vi "Save Preset.vi"(5 "No Oxy?":bool, 6 "Dump Stat":T2, 7 "Preset Name":string, 8 "error in (no error)":errorcluster, 9 "Levels Available":i32, 10 "Levels":T3, 11 "Config":T1) -> (0 "error out":errorcluster, 3 "Config out":T1)   [LabVIEW 2023]
uses:
  <vilib>/Utility/config.llb/Config Data RefNum.ctl
  CTLs/Dump Stat.ctl
  <vilib>/Utility/config.llb/Write Key (I32).vi
  <vilib>/Utility/config.llb/NI_LVConfig.lvlib
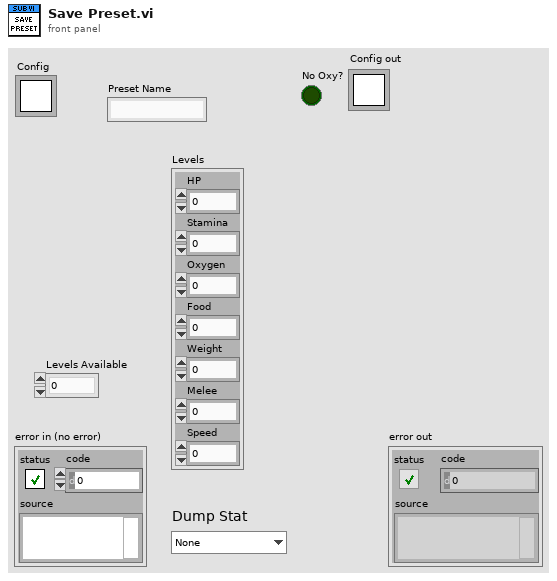
[diagram p1: front panel]
types:
  T1 = typedef "NI_LVConfig.lvlib/Config Data RefNum.ctl" = refnum<k1>
  T2 = typedef "Dump Stat.ctl" = enum16{"None", "HP", "Stamina", "Oxygen", "Food", "Weight", "Melee", "Speed"}
  T3 = cluster{"HP":i32, "Stamina":i32, "Oxygen":i32, "Food":i32, "Weight":i32, "Melee":i32, "Speed":i32}
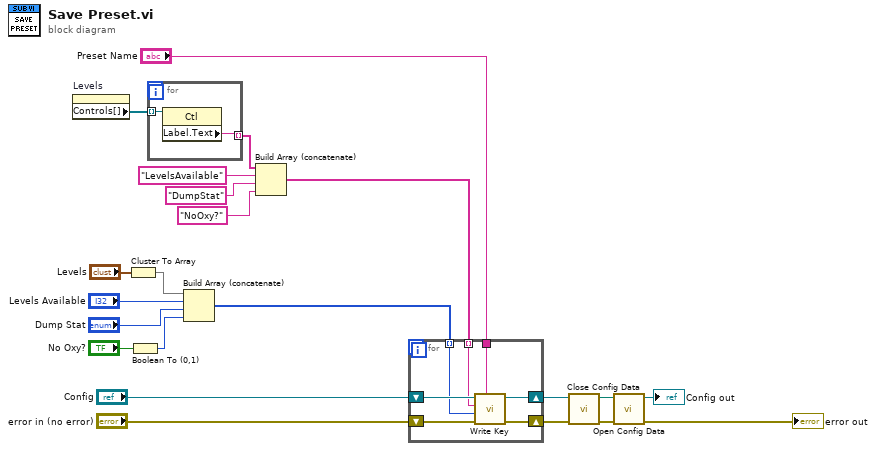
[diagram p0: block diagram]
diagram:
  n1 = property on="Levels" class="Clust (strict)"() -> ("Controls[]"=w22:refnum<vi>[])  [unwired: 2 in, 2 out]
  n2 = Cluster To Array(cluster="Levels") -> (array=w3:i32[])
  n3 = Boolean To (0,1)(Boolean="No Oxy?") -> (0, 1=w6:i16)
  n4 = for {
    tunnel: w22 -> [w24] mode=indexing
    tunnel: [w23] -> w21 mode=indexing
    n5 = property class="Ctl"(reference=w24) -> ("Label.Text"=w23:string)  [unwired: 1 in, 2 out]
  }
  n6 = Build Array (concatenate)(w3, "Levels Available", "Dump Stat", w6) -> (w1:i32[])
  n7 = Build Array (concatenate)(w21, "LevelsAvailable", "DumpStat", "NoOxy?") -> (w2:string[])
  n8 = for {
    tunnel: "Preset Name" -> [w27]
    shift-right: [w29] -> w16
    shift-left: "error in (no error)" -> [w31]
    shift-right: [w30] -> w17
    shift-left: "Config" -> [w28]
    tunnel: w2 -> [w26] mode=indexing
    tunnel: w1 -> [w25] mode=indexing
    n9 = call-poly <vilib>:"Write Key.vi"("section"=w27, "error in (no error)"=w31, "value"=w25, "key"=w26, "refnum"=w28) -> ("error out"=w29:errorcluster, "refnum out"=w30:T1)  [unwired: 4 in, 1 out]
  }
  n10 = call <vilib>:"Close Config Data.vi"("error in (no error)"=w16, "refnum"=w17) -> ("error out"=w14:errorcluster, "file path"=w15:path)  [unwired: 8 in]
  n11 = call <vilib>:"Open Config Data.vi"("error in (no error)"=w14, "configuration file path"=w15) -> ("error out"=→"error out":errorcluster, "refnum"=→"Config out":T1)  [unwired: 7 in, 1 out]
